vi "Learning about Qs.vi"() -> ()   [LabVIEW 2021]
panel:
  out "Iteration":i32
  out "Numeric Indicator":i32
  in  "Numeric Control":i32
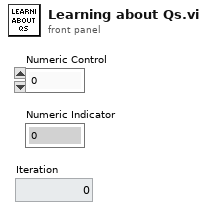
[diagram p1: front panel]
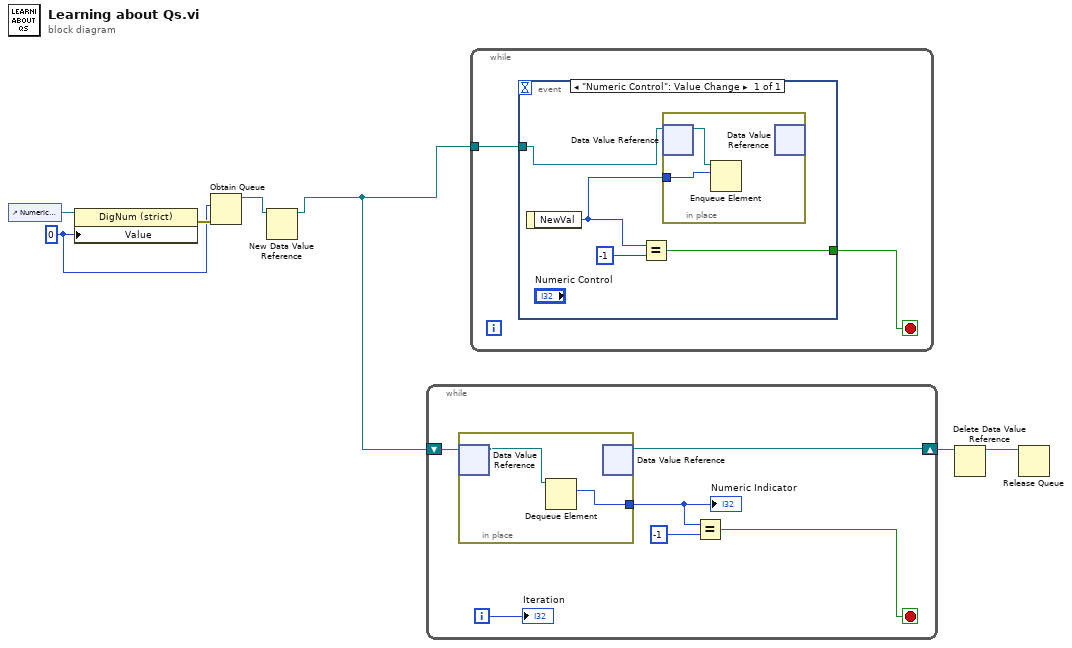
[diagram p0: block diagram]
diagram:
  w5 = 0 ("Value")
  n1 = control-ref of="Numeric Control"() -> (w7:refnum<vi>)
  n2 = property class="DigNum (strict)"(reference=w7, "Value"=w5) -> (error out=w6:errorcluster)  [unwired: 1 in, 1 out]
  n3 = Obtain Queue(element data type=w5, error in (no error)=w6) -> (queue out=w4:refnum<queue>)  [unwired: 3 in, 2 out]
  n4 = New Data Value Reference(data value=w4) -> (data value reference=w2:refnum<data-value>)  [unwired: 1 in, 1 out]
  n5 = while {
    shift-right: [w8] -> w3
    shift-left: w2 -> [w10]
    i -> [w13]
    stop <- w12 stop-if-true
    n6 = in-place {
      in-place-border: [w15] -> w9
      n7 = in-place-dvr #1(w10) -> (w14:refnum<queue>)  [unwired: 1 out]
      n8 = Dequeue Element(queue=w14) -> (element=w15:i32)  [unwired: 2 in, 3 out]
      n9 = in-place-dvr #1() -> (w8:refnum<data-value>)  [unwired: 1 in, 1 out]
    }
    "Numeric Indicator" <- w9
    n10 = Equal?(x=w9, y=-1) -> (x = y?=w12:bool)
    "Iteration" <- w13
  }
  n11 = while {
    tunnel: w2 -> [w16]
    stop <- w17 stop-if-true
    n12 = event shown="[0] \"Numeric Control\": Value Change" {
      selector: _ -> [_]
      dyn-events: _ -> [_]
      timeout: _ -> [_]
      tunnel: w16 -> [w18]
      tunnel: [w20] -> w17
      event "Numeric Control": Value Change {
        n13 = event-data() -> ("NewVal"=w19:i32)  [unwired: 1 in]
        n14 = Equal?(x=w19, y=-1) -> (x = y?=w20:bool)
        n15 = in-place {
          in-place-border: w19 -> [w23]
          n16 = in-place-dvr #2(w18) -> (w22:refnum<queue>)  [unwired: 1 out]
          n17 = Enqueue Element(queue=w22, element=w23) -> ()  [unwired: 2 in, 3 out]
          n18 = in-place-dvr #2() -> ()  [unwired: 1 in, 2 out]
        }
      }
    }
  }
  n19 = Delete Data Value Reference(data value reference=w3) -> (data value=w1:refnum<queue>)  [unwired: 1 in, 1 out]
  n20 = Release Queue(queue=w1) -> ()  [unwired: 2 in, 3 out]
